vi "tcs shm issue Command inject Error LV.vi"(8 "error in (no error)":errorcluster, 11 "command_injectError_Ctl":cluster{"injectError":u8}) -> (0 "error out":errorcluster, 2 "function return":i32, 3 "command_injectError_Ctl out":cluster{"injectError":u8})   [LabVIEW 2016, in "SALLV_tcs.lvlib"]
doc: "int tcs_shm_issueCommand_injectErrorLV(tcs_command_injectErrorLV *command_injectError_Ctl );"
uses:
  SALLV_tcs.lvlib
  SALLV_tcs.so
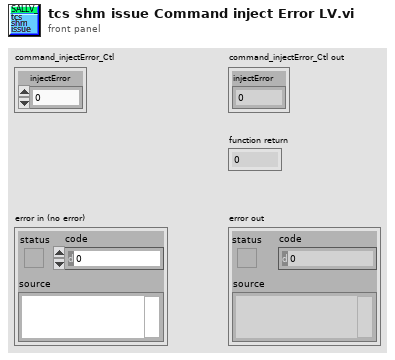
[diagram p1: front panel]
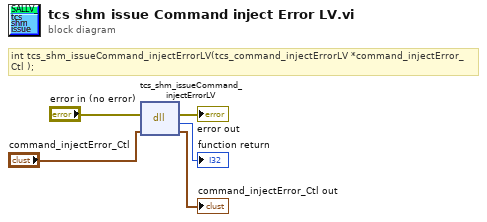
[diagram p0: block diagram]
diagram:
  # "int tcs_shm_issueCommand_injectErrorLV(tcs_command_injectErrorLV *command_injectError_Ctl );"
  n1 = dll-call lib="home/plotz/SALLV_tcs/SALLV_tcs.*" fn="tcs_shm_issueCommand_injectErrorLV"(error in="error in (no error)", "command_injectError_Ctl"="command_injectError_Ctl") -> (error out=→"error out":errorcluster, →"function return":i32, "command_injectError_Ctl"=→"command_injectError_Ctl out":cluster{"injectError":u8})  [unwired: 2 in, 1 out]
